vi "Teleop.vi"(10 "Match Info":T1={"Autonomous Elapsed Seconds"=0.0, "TeleOp Elapsed Seconds"=0.0, "Disabled Elapsed Seconds"=0.0, "Visited Autonomous"=FALSE, "Visited TeleOp"=FALSE, "Visited Disabled"=FALSE, "Autonomous Settings"={"Autonomous Style"=enum."Independent", "VI Refnum"=refnum}}, 11 "Call Context":T2) -> ()   [LabVIEW 2017]
doc: "This VI is called for each TeleOp packet received from the DS where the robot is not disabled. It is often used to read from the joysticks and update I/O or to update setpoints for timed control loops. It should complete and return within 20 milliseconds or it may miss DS packets."
uses:
  <vilib>/Rock Robotics/Network Tables/NT Read Boolean.vi
  <vilib>/Rock Robotics/WPI/Solenoid/WPI_SolenoidValue.ctl
  <vilib>/Rock Robotics/WPI/Solenoid/WPI_SolenoidSetEnum.vi
  Sling_MN_01/Global 1.vi
  <vilib>/Rock Robotics/WPI/ThirdParty/Phoenix-LabVIEW/Motor Controller/Controls/CTRE_Phoenix_MotorControl_ControlMode.ctl
  <vilib>/Rock Robotics/Network Tables/NT Write Numeric Array.vi
  <vilib>/Rock Robotics/Network Tables/NT Read Number.vi
  <vilib>/Rock Robotics/Network Tables/NT Write Boolean Array.vi
  <vilib>/Rock Robotics/WPI/Ultrasonic/WPI_SonarSRF04DigitalRefNum Registry Get.vi
  <vilib>/Rock Robotics/WPI/DriverStation/WPI_DriverStationMatch Info.ctl
  <vilib>/Rock Robotics/WPI/DriverStation/WPI_DriverStationDerivedRobotMode.ctl
panel:
  out "all currents (A)[3]":dbl
  out "all currents (A)[2]":dbl
  out "all currents (A)[1]":dbl
  out "all currents (A)[0]":dbl
  in  "buttonsafety 2":bool
  in  "buttonsafety":bool
  out "positions":dbl
  out "Sample Slider 0":dbl(slide) scale=0.0..5.0
  out "Sample Boolean 1":bool
  out "Sample Boolean 0":bool
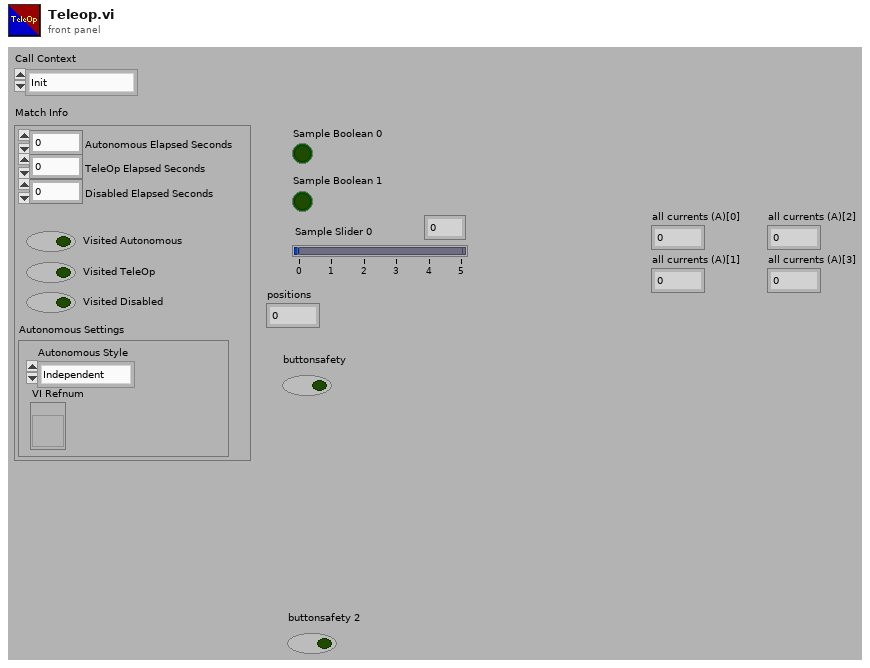
[diagram p1: front panel]
types:
  T1 = typedef "WPI_DriverStationMatch Info.ctl" = cluster{"Autonomous Elapsed Seconds":dbl, "TeleOp Elapsed Seconds":dbl, "Disabled Elapsed Seconds":dbl, "Visited Autonomous":bool, "Visited TeleOp":bool, "Visited Disabled":bool, "Autonomous Settings":cluster{"Autonomous Style":enum16{"Iterative", "Independent"}, "VI Refnum":refnum<vi>}}
  T2 = typedef "WPI_DriverStationDerivedRobotMode.ctl" = enum16{"Init", "Execute", "Stop"}
  T3 = typedef "CTRE_Phoenix_MotorControl_ControlMode.ctl" = u16
  T4 = typedef "WPI_SolenoidValue.ctl" = enum16{"Off", "On", "Forward", "Reverse"}
  T5 = typedef "WPI_JoystickDevRef.ctl" = cluster{"Device":T6}
  T6 = typedef "WPI_JoystickDeviceEnum.ctl" = enum16{"USB 0", "USB 1", "USB 2", "USB 3", "USB 4", "USB 5"}
  T7 = cluster{"Buttons[0]":bool, "Buttons[1]":bool, "Buttons[2]":bool, "Buttons[3]":bool, "Buttons[4]":bool, "Buttons[5]":bool, "Buttons[6]":bool, "Buttons[7]":bool, "Buttons[8]":bool}
  T8 = cluster{"POVs[0]":i16, "POVs[1]":i16, "POVs[2]":i16, "POVs[3]":i16, "POVs[4]":i16, "POVs[5]":i16, "POVs[6]":i16, "POVs[7]":i16, "POVs[8]":i16}
  T9 = cluster{"Axes[0]":dbl, "Axes[1]":dbl, "Axes[2]":dbl, "Axes[3]":dbl, "Axes[4]":dbl, "Axes[5]":dbl, "Axes[6]":dbl, "Axes[7]":dbl, "Axes[8]":dbl}
  T10 = typedef "WPI_SolenoidDevRef.ctl" = cluster{"DevStatus":errorcluster, "Pneumatics Control Module":u8, "Forward Solenoid Channel":T11, "Reverse Solenoid Channel":T11}
  T11 = typedef "WPI_SolenoidChannel.ctl" = enum8{"Solenoid 0", "Solenoid 1", "Solenoid 2", "Solenoid 3", "Solenoid 4", "Solenoid 5", "Solenoid 6", "Solenoid 7", "Invalid"}
  T12 = cluster{"all currents (A)[0]":dbl, "all currents (A)[1]":dbl, "all currents (A)[2]":dbl, "all currents (A)[3]":dbl, "all currents (A)[4]":dbl, "all currents (A)[5]":dbl, "all currents (A)[6]":dbl, "all currents (A)[7]":dbl, "all currents (A)[8]":dbl}
  T13 = typedef "WPI_MotorControlDeviceRef.ctl" = cluster{"DeviceStatus":errorcluster, "Type":T14, "PWM":cluster{"PWM Channel":T15, "DeadBand":T16}, "CAN":cluster{"Device Number":u8, "SetOutput VI Ref":variant, "GetOutput VI Ref":variant, "Enable VI Ref":variant, "Disable VI Ref":variant, "Data":variant}, "Invert":bool, "DIO PWM":cluster{"PWM \"Enable\" Channel":T15, "DIOChannel":T17, "PWM Rate":dbl}}
  T14 = typedef "WPI_MotorControlType.ctl" = enum16{"PWM", "CAN", "DIO PWM"}
  T15 = typedef "FPGA_DIOPWMChannel.ctl" = enum8{"PWM 0", "PWM 1", "PWM 2", "PWM 3", "PWM 4", "PWM 5", "PWM 6", "PWM 7", "PWM 8", "PWM 9", "PWM MXP 0", "PWM MXP 1", "PWM MXP 2", "PWM MXP 3", "PWM MXP 4", "PWM MXP 5", "PWM MXP 6", "PWM MXP 7", "PWM MXP 8", "PWM MXP 9", "Invalid"}
  T16 = typedef "WPI_PWMDeadband.ctl" = cluster{"Name":string, "maxPositivePwm":i32, "minPositivePwm":i32, "centerPwm":i32, "maxNegativePwm":i32, "minNegativePwm":i32, "angularRange":u16}
  T17 = typedef "FPGA_DIOChannel.ctl" = enum8{"DIO 0", "DIO 1", "DIO 2", "DIO 3", "DIO 4", "DIO 5", "DIO 6", "DIO 7", "DIO 8", "DIO 9", "DIO MXP 0", "DIO MXP 1", "DIO MXP 2", "DIO MXP 3", "DIO MXP 4", "DIO MXP 5", "DIO MXP 6", "DIO MXP 7", "DIO MXP 8", "DIO MXP 9", "DIO MXP 10", "DIO MXP 11", "DIO MXP 12", "DIO MXP 13", "DIO MXP 14", "DIO MXP 15", "SPI Port CS1", "SPI Port CS2", "SPI Port CS3", "SPI Port MISO", "SPI Port MOSI", "Invalid"}
  T18 = typedef "WPI_UltrasonicDeviceRef.ctl" = cluster{"DevStatus":errorcluster, "Ping Channel":T17, "Echo Channel":T17, "CntIndex":T19}
  T19 = typedef "FPGA_CounterCtrSystemIndex.ctl" = enum8{"Ctr 0", "Ctr 1", "Ctr 2", "Ctr 3", "Ctr 4", "Ctr 5", "Ctr 6", "Ctr 7", "Invalid"}
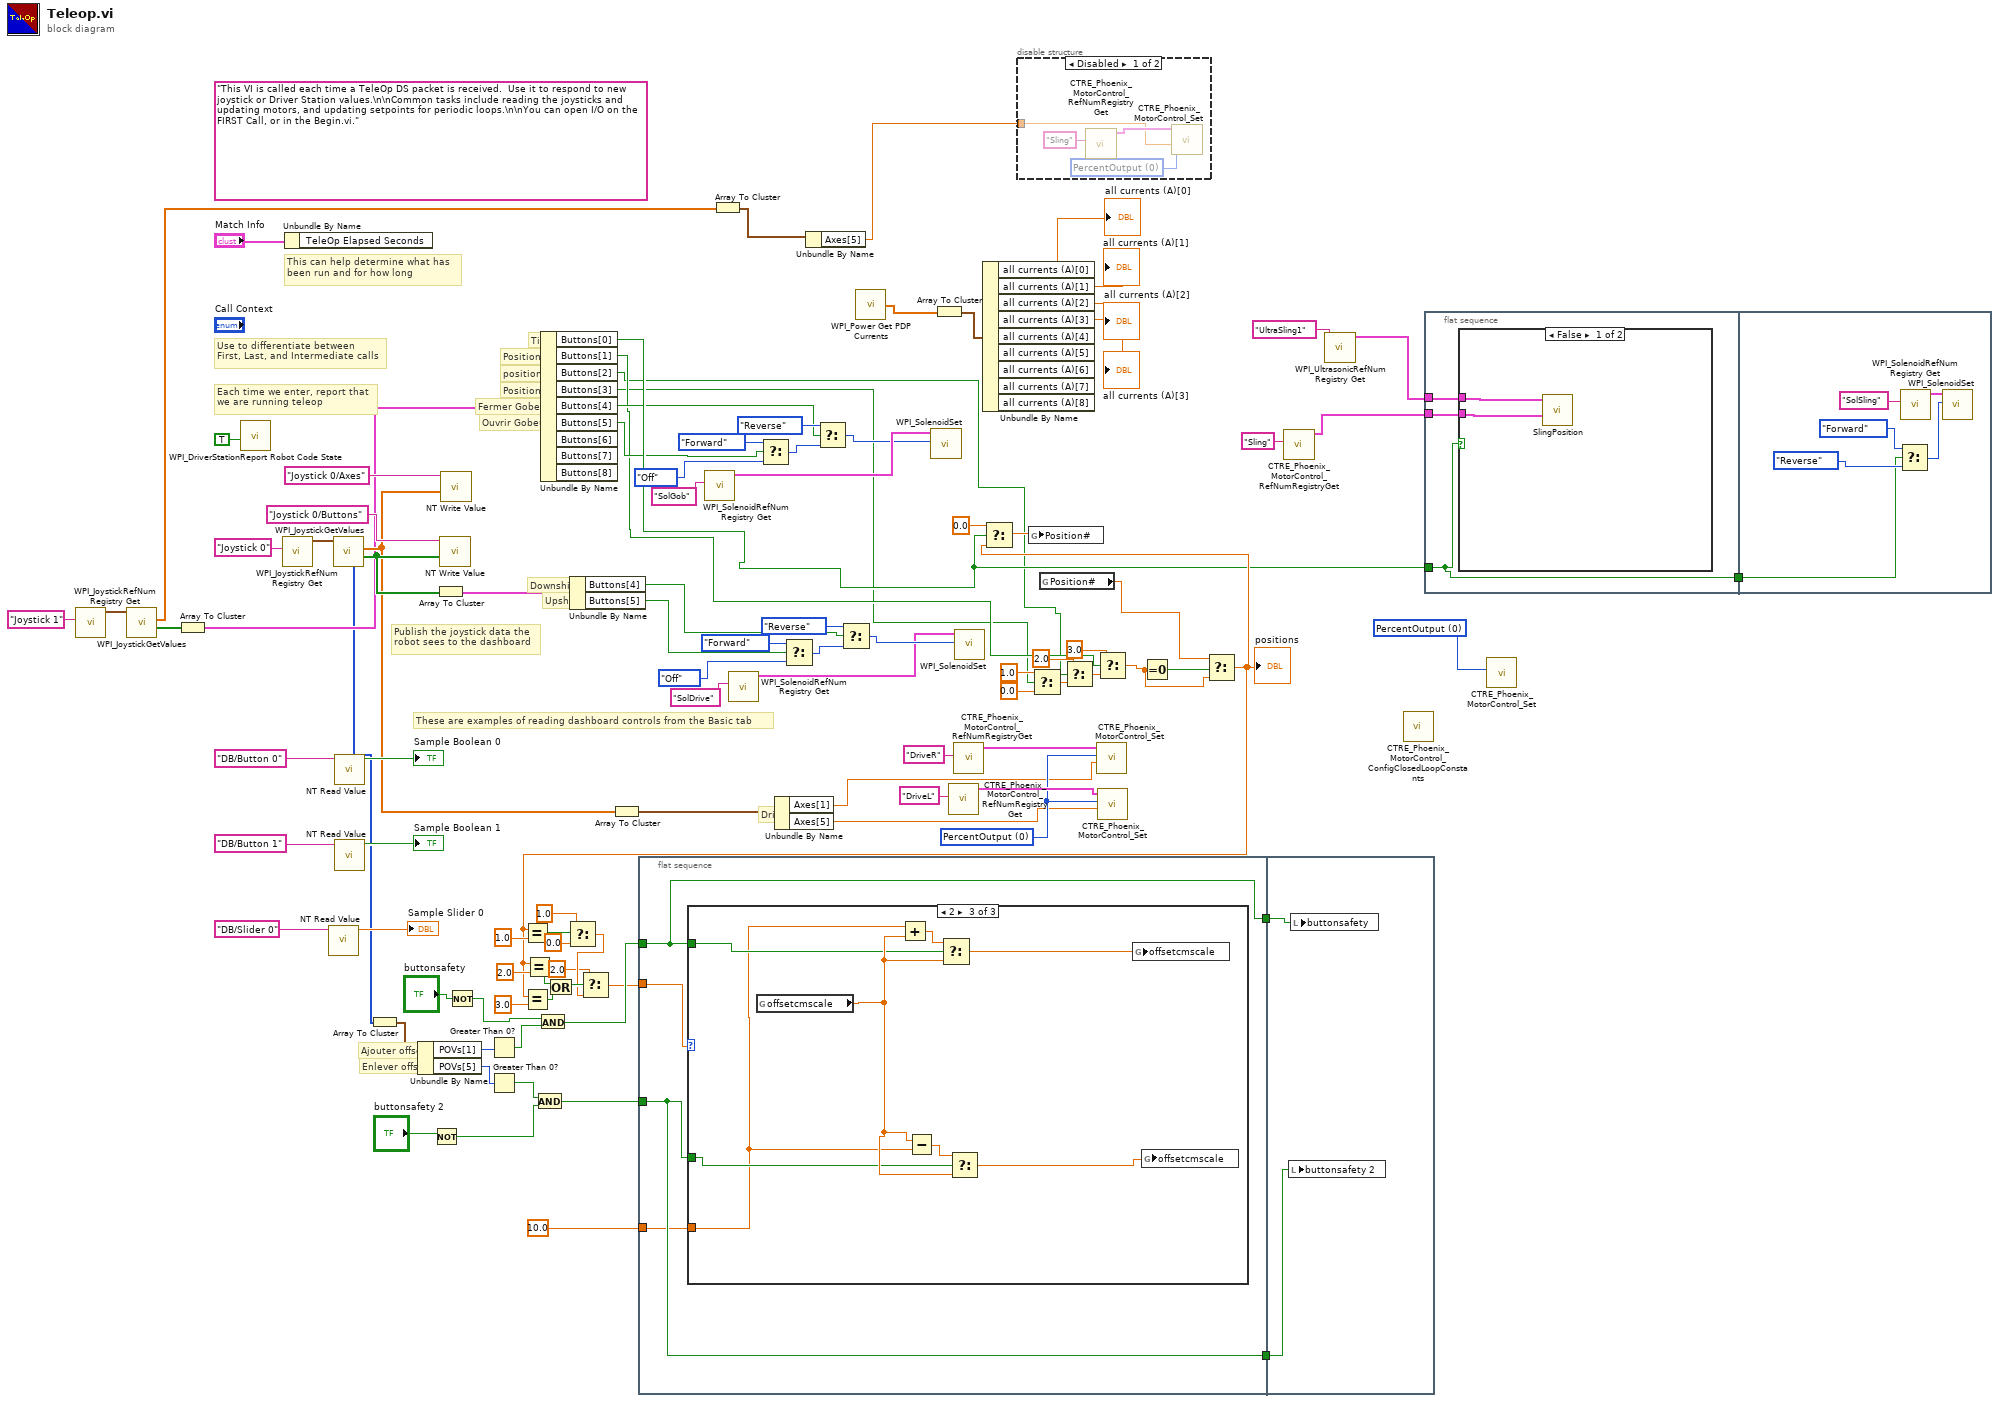
[diagram p0: block diagram]
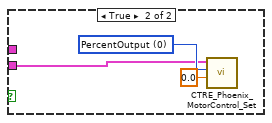
[diagram p3: hidden frame]
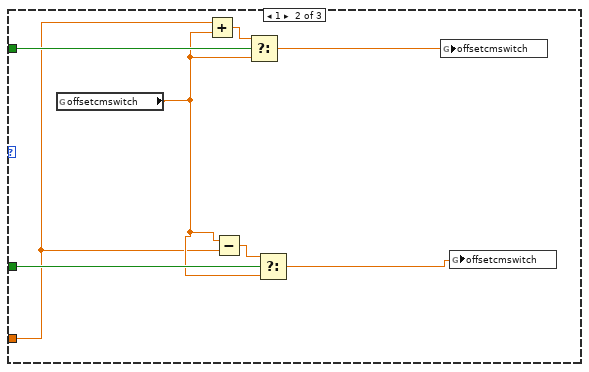
[diagram p5: hidden frame]
diagram:
  w1 = T3 0 items=["PercentOutput"=0, "Position"=1, "Velocity"=2, "Current"=3, "Follower"=5, "MotionProfile"=6, "MotionMagic"=7, "MotionMagicArc"=8, "MotionProfileArc"=10, "Disabled"=15] ("Control Mode")
  w61 = T3 0 items=["PercentOutput"=0, "Position"=1, "Velocity"=2, "Current"=3, "Follower"=5, "MotionProfile"=6, "MotionMagic"=7, "MotionMagicArc"=8, "MotionProfileArc"=10, "Disabled"=15] ("Control Mode")
  (unwired) "This VI is called each time a TeleOp DS packet is received.  Use it to respond to new joystick or Driver Station values.\n\nCommon tasks include reading the joysticks and updating motors, and updating setpoints for periodic loops.\n\nYou can open I/O on the FIRST Call, or in the Begin.vi."
  # "Enlever offset"
  # "Ajouter offset"
  # "Drive"
  # "Upshift"
  # "Downshift"
  # "Ouvrir Gobeur"
  # "Fermer Gobeur"
  # "Position 1"
  # "position 2"
  # "Position 3"
  # "Tirer"
  # "These are examples of reading dashboard controls from the Basic tab"
  # "Publish the joystick data the\nrobot sees to the dashboard"
  # "Each time we enter, report that\nwe are running teleop"
  # "Use to differentiate between\nFirst, Last, and Intermediate calls"
  # "This can help determine what has\nbeen run and for how long"
  n1 = call <vilib>:"WPI_JoystickRefNum Registry Get.vi"("refnum name"="Joystick 1") -> ("JoystickDevRef"=w58:T5)  [unwired: 1 in, 9 out]
  n2 = call <vilib>:"WPI_JoystickGetValues.vi"("JoystickDevRef"=w58) -> ("Buttons"=w56:bool[], "Axes"=w16:dbl[])  [unwired: 6 in, 3 out]
  n3 = Array To Cluster(array=w56) -> (cluster=w55:T7)
  n4 = call <vilib>:"WPI_DriverStationReport Robot Code State.vi"("TeleOp"=TRUE ("Autonomous")) -> ()  [unwired: 10 in, 1 out]
  n5 = call <vilib>:"WPI_JoystickRefNum Registry Get.vi"("refnum name"="Joystick 0") -> ("JoystickDevRef"=w101:T5)  [unwired: 1 in, 9 out]
  n6 = Unbundle By Name("Match Info") -> ()  [unwired: 1 out]
  n7 = call-poly <vilib>:"NT Read Value.vi"("Name"="DB/Slider 0" ("refnum name")) -> ("Numeric"=→"Sample Slider 0":dbl)  [unwired: 9 in, 1 out]
  n8 = call <vilib>:"WPI_JoystickGetValues.vi"("JoystickDevRef"=w101) -> ("Buttons"=w91:bool[], "Axes"=w70:dbl[], "POVs"=w54:i16[])  [unwired: 6 in, 2 out]
  n9 = call-poly <vilib>:"NT Read Value.vi"("Name"="DB/Button 0" ("refnum name")) -> ("Boolean"=→"Sample Boolean 0":bool)  [unwired: 9 in, 1 out]
  n10 = call-poly <vilib>:"NT Read Value.vi"("Name"="DB/Button 1" ("refnum name")) -> ("Boolean"=→"Sample Boolean 1":bool)  [unwired: 9 in, 1 out]
  n11 = Array To Cluster(array=w54) -> (cluster=w53:T8)
  n12 = Unbundle By Name(w53) -> ("POVs[1]"=w52:i16, "POVs[5]"=w51:i16)
  n13 = Not(x="buttonsafety 2") -> (.not. x?=w47:bool)
  n14 = Array To Cluster(array=w91) -> (cluster=w90:T7)
  n15 = call-poly <vilib>:"NT Write Value.vi"("Boolean Array"=w91, "Name"="Joystick 0/Buttons") -> ()  [unwired: 9 in, 1 out]
  n16 = call-poly <vilib>:"NT Write Value.vi"("Numeric Array"=w70, "Name"="Joystick 0/Axes") -> ()  [unwired: 9 in, 1 out]
  n17 = Not(x="buttonsafety") -> (.not. x?=w45:bool)
  n18 = Greater Than 0?(x=w52) -> (x > 0?=w46:bool)
  n19 = Greater Than 0?(x=w51) -> (x > 0?=w48:bool)
  n20 = And(x=w48, y=w47) -> (x .and. y?=w44:bool)
  n21 = And(x=w45, y=w46) -> (x .and. y?=w43:bool)
  n22 = Unbundle By Name(w55) -> ("Buttons[0]"=w7:bool, "Buttons[1]"=w4:bool, "Buttons[2]"=w3:bool, "Buttons[3]"=w2:bool, "Buttons[4]"=w6:bool, "Buttons[5]"=w5:bool)  [unwired: 3 out]
  n23 = Unbundle By Name(w90) -> ("Buttons[4]"=w88:bool, "Buttons[5]"=w87:bool)
  n24 = Array To Cluster(array=w70) -> (cluster=w69:T9)
  n25 = flat-sequence {
    tunnel: w44 -> [w106]
    tunnel: w43 -> [w105]
    tunnel: w31 -> [w107]
    tunnel: [w106] -> w30
    tunnel: [w105] -> w29
    tunnel: 10.0 ("x") -> [w104]
    tunnel: w30 -> [w125]
    tunnel: w29 -> [w124]
    frame #0 {
      n26 = case shown="2" w107 {
        tunnel: w106 -> [_ w115 w117]
        tunnel: w105 -> [_ w114 w118]
        tunnel: w104 -> [_ w110 w116]
        frame 0, Default {
        }
        frame 1 {
          n27 = global read "Global 1.vi" "offsetcmswitch"() -> (w111:dbl)
          n28 = Add(x=w110, y=w111) -> (x+y=w113:dbl)
          n29 = Subtract(x=w111, y=w110) -> (x-y=w112:dbl)
          n30 = Select(t=w113, s=w114, f=w111) -> (s? t:f=w109:dbl)
          n31 = Select(t=w112, s=w115, f=w111) -> (s? t:f=w108:dbl)
          n32 = global write "Global 1.vi" "offsetcmswitch"(w109) -> ()
          n33 = global write "Global 1.vi" "offsetcmswitch"(w108) -> ()
        }
        frame 2 {
          n34 = global read "Global 1.vi" "offsetcmscale"() -> (w121:dbl)
          n35 = Add(x=w116, y=w121) -> (x+y=w123:dbl)
          n36 = Subtract(x=w121, y=w116) -> (x-y=w122:dbl)
          n37 = Select(t=w123, s=w118, f=w121) -> (s? t:f=w120:dbl)
          n38 = Select(t=w122, s=w117, f=w121) -> (s? t:f=w119:dbl)
          n39 = global write "Global 1.vi" "offsetcmscale"(w120) -> ()
          n40 = global write "Global 1.vi" "offsetcmscale"(w119) -> ()
        }
      }
    }
    frame #1 {
      n41 = local write "buttonsafety 2"(w125) -> ()
      n42 = local write "buttonsafety"(w124) -> ()
    }
  }
  n43 = call <vilib>:"WPI_SolenoidRefNum Registry Get.vi"("refnum name"="SolGob") -> ("SolenoidDevRef"=w24:T10)  [unwired: 9 in, 1 out]
  n44 = Array To Cluster(array=w16) -> (cluster=w15:T9)
  n45 = call <vilib>:"WPI_SolenoidRefNum Registry Get.vi"("refnum name"="SolDrive") -> ("SolenoidDevRef"=w82:T10)  [unwired: 9 in, 1 out]
  n46 = Select(t=WPI_SolenoidValue."Forward", s=w5, f=WPI_SolenoidValue."Off" ("Value")) -> (s? t:f=w19:T4)
  n47 = Unbundle By Name(w69) -> ("Axes[1]"=w60:dbl, "Axes[5]"=w59:dbl)
  n48 = Select(t=WPI_SolenoidValue."Forward", s=w87, f=WPI_SolenoidValue."Off" ("Value")) -> (s? t:f=w89:T4)
  n49 = Unbundle By Name(w15) -> ("Axes[5]"=w14:dbl)
  n50 = Select(t=WPI_SolenoidValue."Reverse", s=w6, f=w19) -> (s? t:f=w20:T4)
  n51 = Select(t=WPI_SolenoidValue."Reverse", s=w88, f=w89) -> (s? t:f=w86:T4)
  n52 = call <vilib>:"WPI_Power Get PDP Currents.vi"() -> ("all currents (A)"=w13:dbl[])  [unwired: 13 in, 2 out]
  n53 = call-poly <vilib>:"WPI_SolenoidSet.vi"("Value"=w20, "SolenoidDevRef"=w24) -> ()  [unwired: 8 in, 2 out]
  n54 = Array To Cluster(array=w13) -> (cluster=w12:T12)
  n55 = call "CTRE_Phoenix_MotorControl_RefNumRegistryGet.vi"("refnum name"="DriveL") -> ("PhoenixMotorControlDevRef"=w62:T13)  [unwired: 9 in, 1 out]
  n56 = call "CTRE_Phoenix_MotorControl_RefNumRegistryGet.vi"("refnum name"="DriveR") -> ("PhoenixMotorControlDevRef"=w63:T13)  [unwired: 9 in, 1 out]
  n57 = call-poly <vilib>:"WPI_SolenoidSet.vi"("Value"=w86, "SolenoidDevRef"=w82) -> ()  [unwired: 8 in, 2 out]
  n58 = Unbundle By Name(w12) -> ("all currents (A)[0]"=→"all currents (A)[0]":dbl, "all currents (A)[1]"=→"all currents (A)[1]":dbl, "all currents (A)[2]"=→"all currents (A)[2]":dbl, "all currents (A)[3]"=→"all currents (A)[3]":dbl)  [unwired: 5 out]
  n59 = disable-structure shown="Disabled" {
    disable-tunnel: w14 -> [w126 _]
    frame Disabled {
      w127 = T3 0 items=["PercentOutput"=0, "Position"=1, "Velocity"=2, "Current"=3, "Follower"=5, "MotionProfile"=6, "MotionMagic"=7, "MotionMagicArc"=8, "MotionProfileArc"=10, "Disabled"=15] ("Control Mode")
      n60 = call "CTRE_Phoenix_MotorControl_RefNumRegistryGet.vi"("refnum name"="Sling") -> ("PhoenixMotorControlDevRef"=w128:T13)  [unwired: 9 in, 1 out]
      n61 = call "CTRE_Phoenix_MotorControl_Set.vi"("Output"=w126, "Control Mode"=w127, "PhoenixMotorControlDevRef"=w128) -> ()  [unwired: 7 in, 2 out]
    }
    frame Enabled {
    }
  }
  n62 = Select(t=1.0, s=w2, f=0.0) -> (s? t:f=w79:dbl)
  n63 = global read "Global 1.vi" "Position#"() -> (w68:dbl)
  n64 = Select(t=2.0, s=w3, f=w79) -> (s? t:f=w78:dbl)
  n65 = call "CTRE_Phoenix_MotorControl_Set.vi"("Output"=w60, "Control Mode"=w61, "PhoenixMotorControlDevRef"=w63) -> ()  [unwired: 7 in, 2 out]
  n66 = Select(t=3.0, s=w4, f=w78) -> (s? t:f=w72:dbl)
  n67 = call "CTRE_Phoenix_MotorControl_Set.vi"("Output"=w59, "Control Mode"=w61, "PhoenixMotorControlDevRef"=w62) -> ()  [unwired: 7 in, 2 out]
  n68 = Equal To 0?(x=w72) -> (x = 0?=w73:bool)
  n69 = Select(t=w68, s=w73, f=w72) -> (s? t:f=w27:dbl)
  "positions" <- w27
  n70 = Equal?(x=w27, y=1.0) -> (x = y?=w37:bool)
  n71 = Equal?(x=w27, y=3.0) -> (x = y?=w38:bool)
  n72 = Equal?(x=w27, y=2.0) -> (x = y?=w39:bool)
  n73 = Or(x=w39, y=w38) -> (x .or. y?=w34:bool)
  n74 = Select(t=1.0, s=w37, f=0.0) -> (s? t:f=w33:dbl)
  n75 = Select(t=2.0, s=w34, f=w33) -> (s? t:f=w31:dbl)
  n76 = Select(t=0.0, s=w7, f=w27) -> (s? t:f=w67:dbl)
  n77 = global write "Global 1.vi" "Position#"(w67) -> ()
  n78 = call "CTRE_Phoenix_MotorControl_RefNumRegistryGet.vi"("refnum name"="Sling") -> ("PhoenixMotorControlDevRef"=w18:T13)  [unwired: 9 in, 1 out]
  n79 = call-poly <vilib>:"WPI_UltrasonicRefNum Registry Get.vi"("refnum name"="UltraSling1") -> ("SonarSRF04DevRef"=w17:T18)  [unwired: 9 in, 1 out]
  n80 = call <vilib>:"CTRE_Phoenix_MotorControl_ConfigClosedLoopConstants.vi"() -> ()  [unwired: 14 in, 2 out]
  n81 = flat-sequence {
    tunnel: w7 -> [w132]
    tunnel: [w132] -> w26
    tunnel: w18 -> [w131]
    tunnel: w17 -> [w130]
    tunnel: w26 -> [w138]
    frame #0 {
      n82 = case shown="False" w132 {
        tunnel: w131 -> [w134 w136]
        tunnel: w130 -> [w133 _]
        frame False {
          n83 = call "SlingPosition.vi"("PhoenixMotorControlDevRef"=w134, "SonarSRF04DevRef"=w133) -> ()  [unwired: 9 in, 1 out]
        }
        frame True {
          w137 = T3 0 items=["PercentOutput"=0, "Position"=1, "Velocity"=2, "Current"=3, "Follower"=5, "MotionProfile"=6, "MotionMagic"=7, "MotionMagicArc"=8, "MotionProfileArc"=10, "Disabled"=15] ("Control Mode")
          n84 = call "CTRE_Phoenix_MotorControl_Set.vi"("Output"=0.0, "Control Mode"=w137, "PhoenixMotorControlDevRef"=w136) -> ()  [unwired: 7 in, 2 out]
        }
      }
    }
    frame #1 {
      n85 = Select(t=WPI_SolenoidValue."Forward", s=w138, f=WPI_SolenoidValue."Reverse" ("Value")) -> (s? t:f=w142:T4)
      n86 = call <vilib>:"WPI_SolenoidRefNum Registry Get.vi"("refnum name"="SolSling") -> ("SolenoidDevRef"=w143:T10)  [unwired: 9 in, 1 out]
      n87 = call-poly <vilib>:"WPI_SolenoidSet.vi"("Value"=w142, "SolenoidDevRef"=w143) -> ()  [unwired: 8 in, 2 out]
    }
  }
  n88 = call "CTRE_Phoenix_MotorControl_Set.vi"("Control Mode"=w1) -> ()  [unwired: 9 in, 2 out]
